vi "Hardware in the Loop - Clear Unfinished Shot.vi"(8 "error in":errorcluster, 11 "Configuration Cluster":T1={"Name"="Default Settings", "IP"="192.168.0.84", "Control Port"=4220, "Timeout (ms)"=2000, "Continuous Capture Port (Multiplexed)"=4210, "Start HIL Shot Port"=53999, "AWG Upload Port (Multiplexed)"=54201, "Download Captured Data Port (Multiplexed)"=53000, "Module Slots"=2, "Module Configurations"=[{"Name"="ACQ 425 ELF", "Position"="192.168.0.84", "Module Type"=enum."Analog In Module", "Control Port"=4221, "Timeout (ms)"=2000, "Channels"=16}, {"Name"="AO 424 ELF", "Position"="192.168.0.84", "Module Type"=enum."Analog Out Module", "Control Port"=4222, "Timeout (ms)"=2000, "Channels"=16}]}) -> (0 "error out":errorcluster, 2 "Ready":bool=TRUE)   [LabVIEW 2017, in "Communications Library.lvlib"]
doc: "Querries the status of the DTACQ device.\n\nIf the analog out module is busy, a shot is run in order to clear the state. This can occur if a waveform was uploaded but never run, during a previous execution of the software."
uses:
  Communications Library.lvlib
  Typedefs/DTACQ Module Carrier Configuration--Cluster.ctl
  Typedefs/DTACQ Module Configuration--Cluster.ctl
  Typedefs/DTACQ Device Type--Enum.ctl
panel:
  out "millisecond timer":u32
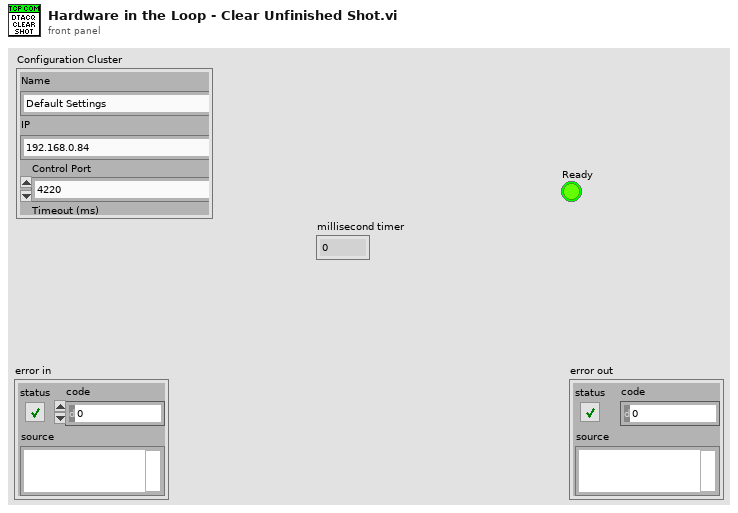
[diagram p1: front panel]
types:
  T1 = typedef "Communications Library.lvlib/DTACQ Module Carrier Configuration--Cluster.ctl" = cluster{"Name":string, "IP":string, "Control Port":i32, "Timeout (ms)":i32, "Continuous Capture Port (Multiplexed)":i32, "Start HIL Shot Port":i32, "AWG Upload Port (Multiplexed)":i32, "Download Captured Data Port (Multiplexed)":i32, "Module Slots":i32, "Module Configurations":T2[]}
  T2 = typedef "Communications Library.lvlib/DTACQ Module Configuration--Cluster.ctl" = cluster{"Name":string, "Position":string, "Module Type":T3, "Control Port":i32, "Timeout (ms)":i32, "Channels":i32}
  T3 = typedef "Communications Library.lvlib/DTACQ Device Type--Enum.ctl" = enum16{"Carrier", "Analog In Module", "Analog Out Module", "Generic Module"}
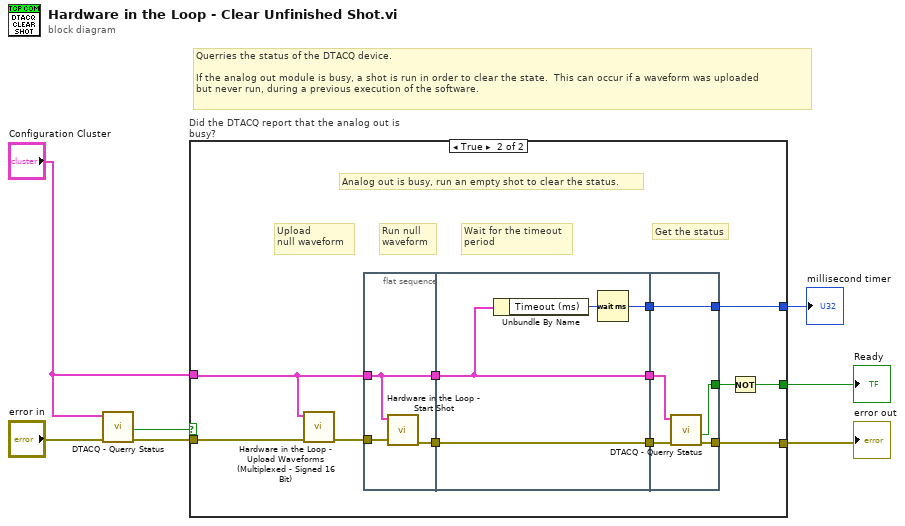
[diagram p0: block diagram]
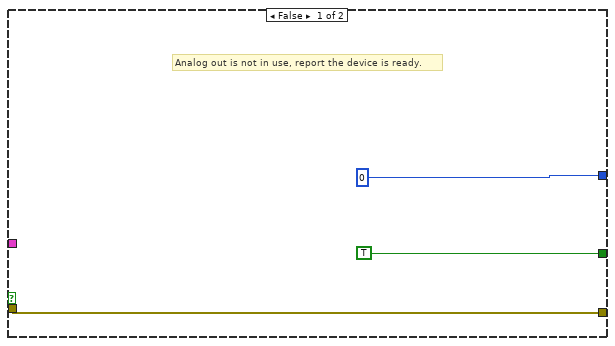
[diagram p2: hidden frame]
diagram:
  # "Querries the status of the DTACQ device.\n\nIf the analog out module is busy, a shot is run in order to clear the state.  This can occur if a waveform was uploaded \nbut never run, during a previous execution of the software."
  n1 = call "DTACQ - Querry Status.vi"("error in"="error in", "Configuration Cluster"="Configuration Cluster") -> ("error out"=w6:errorcluster, "Analog Out Busy"=w7:bool)  [unwired: 6 in, 2 out]
  n2 = case "Did the DTACQ report that the analog out is busy?" shown="True" w7 {
    tunnel: w6 -> [w10 w13]
    tunnel: "Configuration Cluster" -> [_ w11]
    tunnel: [w10 w22] -> w5
    tunnel: [TRUE w21] -> w4
    tunnel: [u32 0 ("millisecond timer value") w20] -> w2
    frame False {
      # "Analog out is not in use, report the device is ready."
    }
    frame True {
      # "Analog out is busy, run an empty shot to clear the status."
      # "Get the status"
      # "Wait for the timeout\nperiod"
      # "Run null \nwaveform"
      # "Upload \nnull waveform"
      n3 = call "Hardware in the Loop - Upload Waveforms (Multiplexed - Signed 16 Bit).vi"("error in"=w13, "Configuration Cluster"=w11) -> ("error out"=w12:errorcluster)  [unwired: 9 in]
      n4 = flat-sequence {
        tunnel: w12 -> [w25]
        tunnel: w11 -> [w23]
        tunnel: [w24] -> w19
        tunnel: [w23] -> w18
        tunnel: [w29] -> w17
        tunnel: w19 -> [w29]
        tunnel: [w28] -> w16
        tunnel: w18 -> [w26]
        tunnel: [w26] -> w15
        tunnel: w17 -> [w34]
        tunnel: [w33] -> w20
        tunnel: w16 -> [w33]
        tunnel: [w32] -> w22
        tunnel: [w31] -> w14
        tunnel: w15 -> [w30]
        frame #0 {
          n5 = call "Hardware in the Loop - Start Shot.vi"("error in"=w25, "Configuration Cluster"=w23) -> ("error out"=w24:errorcluster)  [unwired: 8 in, 1 out]
        }
        frame #1 {
          n6 = Unbundle By Name(w26) -> ("Timeout (ms)"=w27:i32)
          n7 = Wait (ms)(milliseconds to wait=w27) -> (millisecond timer value=w28:u32)
        }
        frame #2 {
          n8 = call "DTACQ - Querry Status.vi"("error in"=w34, "Configuration Cluster"=w30) -> ("error out"=w32:errorcluster, "Analog Out Busy"=w31:bool)  [unwired: 6 in, 2 out]
        }
      }
      n9 = Not(x=w14) -> (.not. x?=w21:bool)
    }
  }
  "error out" <- w5
  "Ready" <- w4
  "millisecond timer" <- w2
